vi "Destroy.vi"(0 "reference":refnum<class "InterfaceNode.lvclass">, 5 "error in (no error)":errorcluster) -> (14 "reference out":refnum<class "InterfaceNode.lvclass">, 19 "error out":errorcluster)   [LabVIEW 2020, in "InterfaceNode.lvclass"]
doc: "Destroys a InterfaceNode object created with a InterfaceNode constructor VI.\n\n[GOOP 2.1]"
uses:
  <resource>/Framework/Providers/Open_GDS/UML/InterfaceNode_class/InterfaceNode.lvclass
  <resource>/Framework/Providers/Open_GDS/UML/ClassNode_class/ClassNode.lvclass
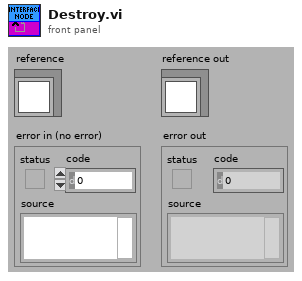
[diagram p1: front panel]
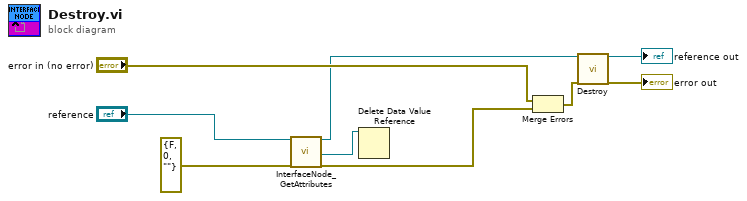
[diagram p0: block diagram]
diagram:
  n1 = call <resource>:"InterfaceNode_GetAttributes.vi"("reference in"="reference", "error in (no error)"=errorcluster {"status"=FALSE, "code"=0, "source"=""}) -> ("reference out"=w7:refnum<class "InterfaceNode.lvclass">, "DataRef"=w5:refnum<data-value>, "error out"=w1:errorcluster)  [unwired: 1 in, 14 out]
  n2 = Delete Data Value Reference(data value reference=w5) -> ()  [unwired: 1 in, 2 out]
  n3 = Merge Errors("error in (no error)", w1) -> (w6:errorcluster)
  n4 = call-parent "Destroy.vi"("reference"=w7, "error in (no error)"=w6) -> ("reference out"=→"reference out":refnum<class "InterfaceNode.lvclass">, "error out"=→"error out":errorcluster)  [unwired: 16 in]
